vi "Configure Efficiency User Define.vi"(4 "D (0: None)":i32(ring) items=["None", "Active Power 1", "Active Power 2", "Active Power 3", "Active Power 4", "Active Power 5", "Active Power 6", "Active Power Sigma A", "Active Power Sigma B", "Active Power Sigma C", "Pm"], 6 "C (0: None)":i32(ring) items=["None", "Active Power 1", "Active Power 2", "Active Power 3", "Active Power 4", "Active Power 5", "Active Power 6", "Active Power Sigma A", "Active Power Sigma B", "Active Power Sigma C", "Pm"], 7 "Define Number (1)":i32=1 min=1 max=2 step=1, 8 "error in (no error)":errorcluster, 9 "B (0: None)":i32(ring) items=["None", "Active Power 1", "Active Power 2", "Active Power 3", "Active Power 4", "Active Power 5", "Active Power 6", "Active Power Sigma A", "Active Power Sigma B", "Active Power Sigma C", "Pm"], 10 "A (0: None)":i32(ring) items=["None", "Active Power 1", "Active Power 2", "Active Power 3", "Active Power 4", "Active Power 5", "Active Power 6", "Active Power Sigma A", "Active Power Sigma B", "Active Power Sigma C", "Pm"], 11 "VISA resource name":refnum<visa-resource-name>) -> (0 "error out":errorcluster, 3 "VISA resource name out":refnum<visa-resource-name>)   [LabVIEW 2021, in "Yokogawa WT1800 Series.lvlib"]
doc: "Create an user define function to use efficiency equation"
uses:
  <instrlib>/Yokogawa WT1800 Series/Yokogawa WT1800 Series.lvlib
panel:
  # "+"
  # "+"
  # "+"
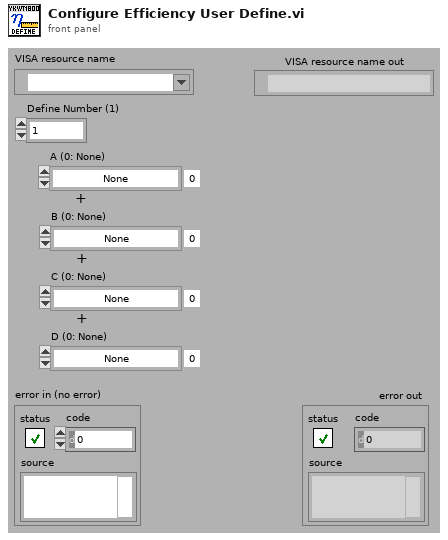
[diagram p1: front panel]
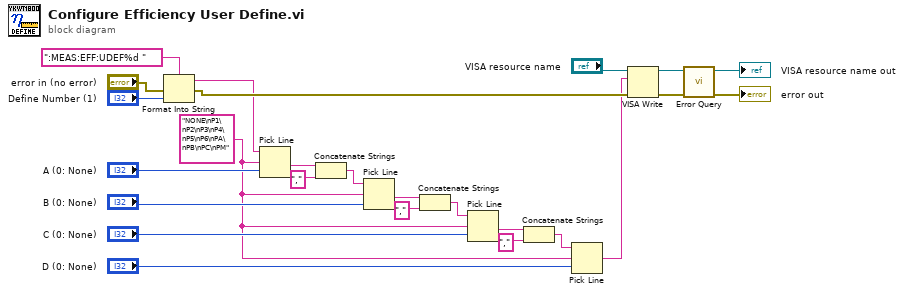
[diagram p0: block diagram]
diagram:
  w11 = "NONE\nP1\nP2\nP3\nP4\nP5\nP6\nPA\nPB\nPC\nPM" ("複数行文字列")
  n1 = Format Into String ("文字列にフォーマット")(format string=":MEAS:EFF:UDEF%d " ("形式文字列"), error in="error in (no error)", "Define Number (1)") -> (resulting string=w16:string, error out=w19:errorcluster)  [unwired: 1 in]
  n2 = Pick Line ("ライン選択")(string ("")=w16, multi-line string=w11, line index="A (0: None)") -> (output string=w4:string)
  n3 = Concatenate Strings(w4, "," ("文字列")) -> (w2:string)
  n4 = Pick Line ("ライン選択")(string ("")=w2, multi-line string=w11, line index="B (0: None)") -> (output string=w3:string)
  n5 = Concatenate Strings(w3, "," ("文字列")) -> (w7:string)
  n6 = Pick Line ("ライン選択")(string ("")=w7, multi-line string=w11, line index="C (0: None)") -> (output string=w1:string)
  n7 = Concatenate Strings(w1, "," ("文字列")) -> (w5:string)
  n8 = Pick Line ("ライン選択")(string ("")=w5, multi-line string=w11, line index="D (0: None)") -> (output string=w10:string)
  n9 = VISA Write ("VISA書き込み")(VISA resource name="VISA resource name", write buffer=w10, error in (no error)=w19) -> (VISA resource name out=w25:refnum<visa-resource-name>, error out=w24:errorcluster)  [unwired: 1 out]
  n10 = call <instrlib>:"Error Query.vi"("error in (no error)"=w24, "VISA resource name"=w25) -> ("error out"=→"error out":errorcluster, "VISA resource name out"=→"VISA resource name out":refnum<visa-resource-name>)  [unwired: 6 in, 2 out]
